vi "shutdown.vi"(8 "error in":errorcluster, 11 "Target Runtime in":refnum<class "PL_Target Runtime.lvclass">) -> (0 "error out":errorcluster)   [LabVIEW 2013, in "PL_Target Runtime.lvclass"]
uses:
  PL_Target Runtime.lvclass
  PL_Target Runtime.lvclass/PL_Target Runtime.ctl
  <vilib>/NI/Tag Bus Module Framework/FPGA manager/methods.ctl
  <vilib>/NI/Tag Bus Module Framework/FPGA manager/FPGA manager.lvlib
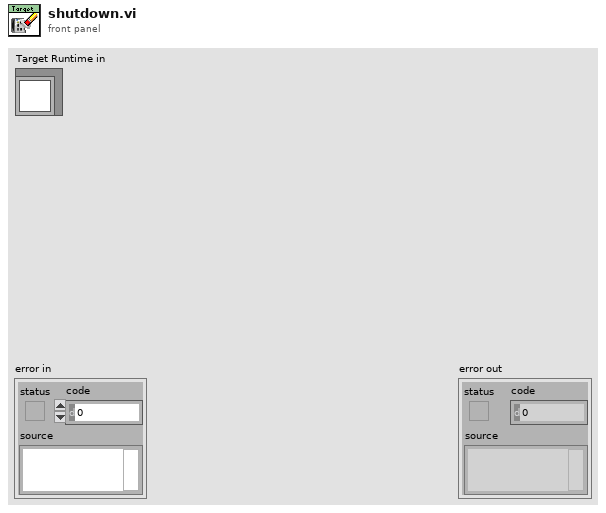
[diagram p1: front panel]
types:
  T1 = typedef "FPGA manager.lvlib/methods.ctl" = enum16{"initialize bitfile", "cache bitfile", "locate bitfile", "close bitfile"}
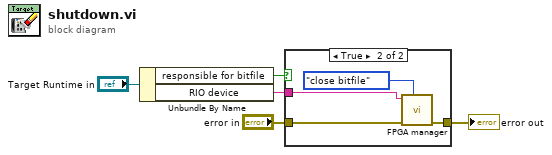
[diagram p0: block diagram]
diagram:
  n1 = Unbundle By Name("Target Runtime in") -> ("responsible for bitfile"=w4:bool, "RIO device"=w1:string)
  n2 = case shown="True" w4 {
    tunnel: "error in" -> [w6 w9]
    tunnel: [w6 w8] -> w2
    tunnel: w1 -> [_ w7]
    frame False {
    }
    frame True {
      n3 = call <vilib>:"FPGA manager.vi"("action"=methods."close bitfile", "error in"=w9, "RIO resource"=w7) -> ("error out"=w8:errorcluster)  [unwired: 6 in, 2 out]
    }
  }
  "error out" <- w2
